vi "Time Stamp To Time String.vi"(7 "Format":string="%Y/%m%d %H:%M:%S%3u", 10 "Time Stamp In":timestamp format="%<%.3X %x>T") -> (2 "String Out":string)   [LabVIEW 2024]
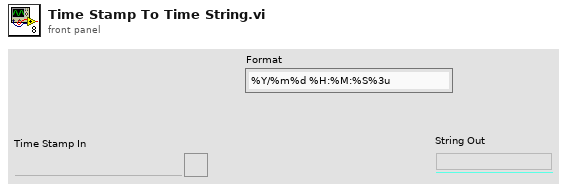
[diagram p1: front panel]
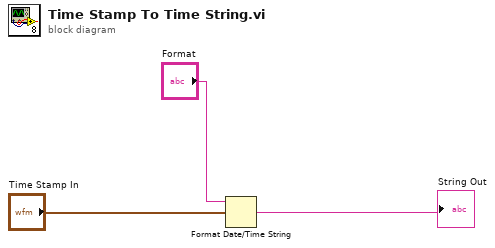
[diagram p0: block diagram]
diagram:
  n1 = Format Date/Time String(time format string (%c)="Format", seconds (now)="Time Stamp In") -> (date/time string=→"String Out":string)  [unwired: 1 in]
